vi "fftw_memcpy_to_cplx.vi"(8 "error in (no error)":errorcluster, 10 "cplx count":i32, 11 "*data_in":u64) -> (0 "error out":errorcluster, 2 "cplx dbl array out":cdb[](array[numeric]), 3 "*data_in (copy)":u64)   [LabVIEW 2020, in "FFTWDLL.lvlib"]
doc: "Copy FFTW cplx double data to LV CDBL array."
uses:
  FFTWDLL.lvlib
  ntdll.dll
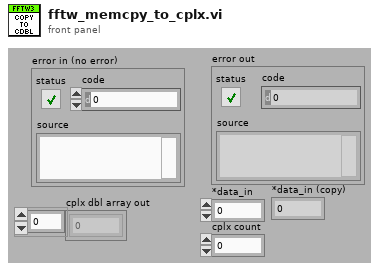
[diagram p1: front panel]
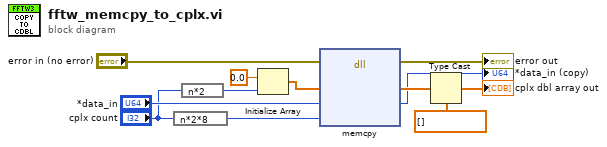
[diagram p0: block diagram]
diagram:
  n1 = expression code="n*2*8"("cplx count") -> (w10:i32)
  n2 = expression code="n*2"("cplx count") -> (w5:i32)
  n3 = Initialize Array(0.0, w5) -> (w8:dbl[])
  n4 = dll-call lib="ntdll.dll" fn="memcpy"(error in="error in (no error)", "dest"=w8, "src"="*data_in", "n"=w10) -> (error out=→"error out":errorcluster, "dest"=w4:dbl[], "src"=→"*data_in (copy)":i64)  [unwired: 4 in, 1 out]
  n5 = Type Cast(type=cdb[] [], x=w4) -> (*(type *) &x=→"cplx dbl array out":cdb[])
